vi "RT - DI Status Change.vi"(6 "DI Index":i32, 8 "Error In":errorcluster, 9 "Last Status":bool, 10 "Current Status":bool, 11 "Message Queue":refnum<queue>) -> (0 "Error Out":errorcluster, 2 "Current Status Out":bool, 3 "dup Message Queue":refnum<queue>)   [LabVIEW 2018]
uses:
  Message Queue/Message Cluster.ctl
  Message Queue/Message.ctl
  Controls/Control Mode.ctl
  Controls/DI Status Message.ctl
  Message Queue/Message Queue.lvlib
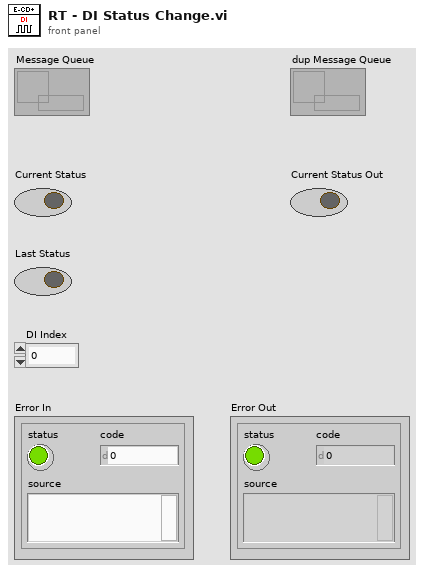
[diagram p1: front panel]
types:
  T1 = typedef "Message Queue.lvlib/Message.ctl" = enum16{"Initialize", "Initialize UI Refs", "Disable Controls", "Enable UI Controls", "Connect RT", "Get Control Mode from RT", "Send Control Mode to UI", "Update Control Mode", "Get Config from RT", "Send Config to UI", "Update Parameters", "Change Parameters", "Calibrate Config", "Update Calibration", "Change Valve State", "Get Valve Status from RT", "Send Valve Status to UI", "Update Valve Status", "Inital UI Values", "Disconnect RT", "Close Connection", "Disconnect UI", "Run Mode", "Stop ALL", "Change Control Mode", "Skid Manual", "Computer Manual", "Step Automated", "Fully Automated", "Reset", "Pumps Command", "Pump State Changed", "Critical Error", "Log-Only Error", "Non-Critical Error", "RT Error", "Update System Status", "Update DI Status", "Clear System Status", "Update Warning", "Clear Warning", "Upate Timeout", "Update Reset Status", "Waiting", "Verify Password", "Manual Cleaning Process", "Update Manual Cleaning Process", "Cal - Body", "Cal - US", "Cal - Update Parameters", "Exit", "---Copy This Frame---"}
  T2 = typedef "Control Mode.ctl" = enum16{"Skid Manual", "Computer Manual", "Step Automated", "Fully Automated"}
  T3 = typedef "DI Status Message.ctl" = cluster{"Message":string, "DI Index #":i32, "Status":bool}
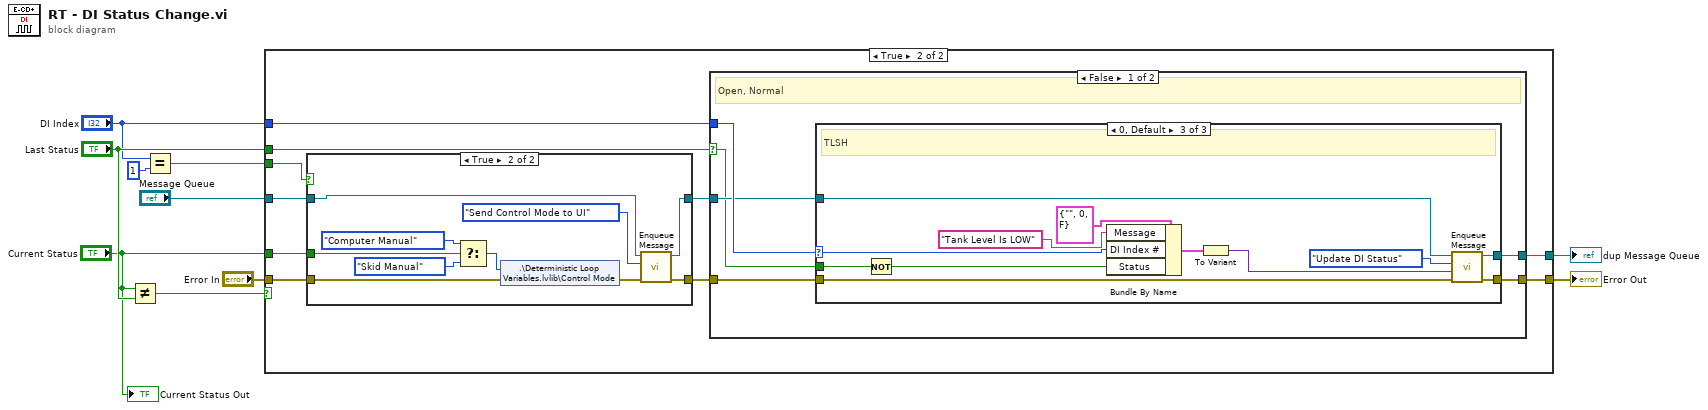
[diagram p0: block diagram]
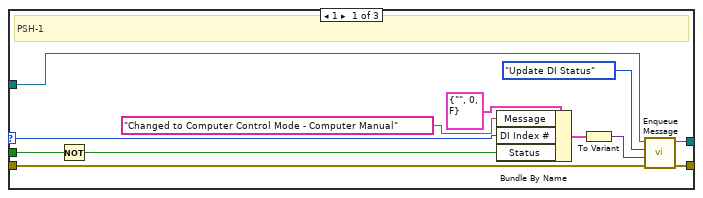
[diagram p4: hidden frame]
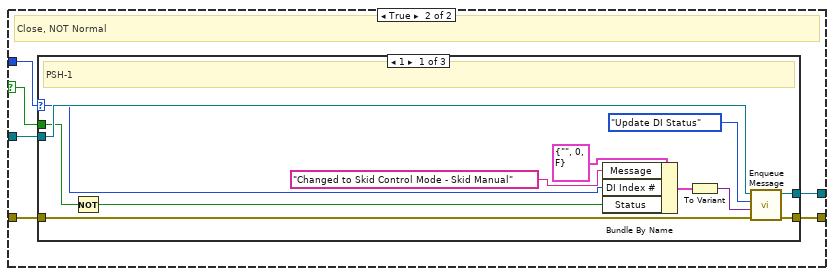
[diagram p6: hidden frame]
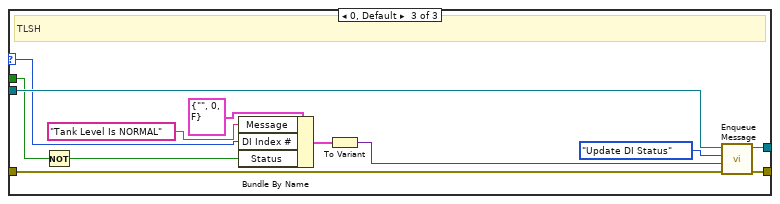
[diagram p8: hidden frame]
diagram:
  n1 = Not Equal?(x="Current Status", y="Last Status") -> (x != y?=w6:bool)
  n2 = Equal?(x="DI Index", y=1) -> (x = y?=w3:bool)
  n3 = case shown="True" w6 {
    tunnel: "Last Status" -> [_ w22]
    tunnel: "DI Index" -> [_ w21]
    tunnel: "Message Queue" -> [w11 w14]
    tunnel: "Error In" -> [w12 w17]
    tunnel: [w12 w20] -> w9
    tunnel: [w11 w19] -> w8
    tunnel: w3 -> [_ w18]
    tunnel: "Current Status" -> [_ w15]
    frame False {
    }
    frame True {
      n4 = case shown="True" w18 {
        tunnel: w17 -> [w24 w30]
        tunnel: [w24 w28] -> w16
        tunnel: w15 -> [_ w34]
        tunnel: w14 -> [w23 w27]
        tunnel: [w23 w26] -> w13
        frame False {
        }
        frame True {
          n5 = Select(t=Control_Mode."Computer Manual" ("Control Mode"), s=w34, f=Control_Mode."Skid Manual") -> (s? t:f=w31:T2)
          n6 = shared-variable ".\\Deterministic Loop Variables.lvlib\\Control Mode"(w31, error in=w30) -> (error out=w29:errorcluster)
          n7 = call "Enqueue Message.vi"("error in (no error)"=w29, "Message"=Message."Send Control Mode to UI", "Message Queue"=w27) -> ("error out"=w28:errorcluster, "dup Message Queue"=w26:refnum<queue>)  [unwired: 7 in]
        }
      }
      n8 = case shown="False" w22 {
        selector: w22 -> [w36 w68]
        tunnel: w13 -> [w39 w71]
        tunnel: w21 -> [w40 w72]
        tunnel: w16 -> [w38 w70]
        tunnel: [w37 w69] -> w20
        tunnel: [w35 w67] -> w19
        frame False {
          # "Open, Normal"
          n9 = case shown="0, Default" w40 {
            selector: w40 -> [w47 _ w61]
            tunnel: w39 -> [w52 w54 w66]
            tunnel: w38 -> [w50 w53 w64]
            tunnel: [w49 w53 w63] -> w37
            tunnel: w36 -> [w46 _ w60]
            tunnel: [w41 w54 w55] -> w35
            frame 1 {
              # "PSH-1"
              n10 = Not(x=w46) -> (.not. x?=w45:bool)
              n11 = Bundle By Name(cluster=T3 {"Message"="", "DI Index #"=0, "Status"=FALSE} ("DI Status Message"), "Message"="Changed to Computer Control Mode - Computer Manual", "DI Index #"=w47, "Status"=w45) -> (w43:T3)
              n12 = To Variant(anything=w43) -> (Variant=w44:variant)
              n13 = call "Enqueue Message.vi"("error in (no error)"=w50, "Message Data"=w44, "Message"=Message."Update DI Status", "Message Queue"=w52) -> ("error out"=w49:errorcluster, "dup Message Queue"=w41:refnum<queue>)  [unwired: 6 in]
            }
            frame 2..22 {
            }
            frame 0, Default {
              # "TLSH"
              n14 = Not(x=w60) -> (.not. x?=w59:bool)
              n15 = Bundle By Name(cluster=T3 {"Message"="", "DI Index #"=0, "Status"=FALSE} ("DI Status Message"), "Message"="Tank Level Is LOW", "DI Index #"=w61, "Status"=w59) -> (w57:T3)
              n16 = To Variant(anything=w57) -> (Variant=w58:variant)
              n17 = call "Enqueue Message.vi"("error in (no error)"=w64, "Message Data"=w58, "Message"=Message."Update DI Status", "Message Queue"=w66) -> ("error out"=w63:errorcluster, "dup Message Queue"=w55:refnum<queue>)  [unwired: 6 in]
            }
          }
        }
        frame True {
          # "Close, NOT Normal"
          n18 = case shown="1" w72 {
            selector: w72 -> [w80 _ w93]
            tunnel: w71 -> [w84 w86 w98]
            tunnel: w70 -> [w74 w85 w96]
            tunnel: [w82 w85 w95] -> w69
            tunnel: w68 -> [w79 _ w92]
            tunnel: [w75 w86 w87] -> w67
            frame 1 {
              # "PSH-1"
              n19 = Not(x=w79) -> (.not. x?=w73:bool)
              n20 = Bundle By Name(cluster=T3 {"Message"="", "DI Index #"=0, "Status"=FALSE} ("DI Status Message"), "Message"="Changed to Skid Control Mode - Skid Manual", "DI Index #"=w80, "Status"=w73) -> (w77:T3)
              n21 = To Variant(anything=w77) -> (Variant=w78:variant)
              n22 = call "Enqueue Message.vi"("error in (no error)"=w74, "Message Data"=w78, "Message"=Message."Update DI Status", "Message Queue"=w84) -> ("error out"=w82:errorcluster, "dup Message Queue"=w75:refnum<queue>)  [unwired: 6 in]
            }
            frame 2..22 {
            }
            frame 0, Default {
              # "TLSH"
              n23 = Not(x=w92) -> (.not. x?=w91:bool)
              n24 = Bundle By Name(cluster=T3 {"Message"="", "DI Index #"=0, "Status"=FALSE} ("DI Status Message"), "Message"="Tank Level Is NORMAL", "DI Index #"=w93, "Status"=w91) -> (w89:T3)
              n25 = To Variant(anything=w89) -> (Variant=w90:variant)
              n26 = call "Enqueue Message.vi"("error in (no error)"=w96, "Message Data"=w90, "Message"=Message."Update DI Status", "Message Queue"=w98) -> ("error out"=w95:errorcluster, "dup Message Queue"=w87:refnum<queue>)  [unwired: 6 in]
            }
          }
        }
      }
    }
  }
  "Error Out" <- w9
  "dup Message Queue" <- w8
  "Current Status Out" <- "Current Status"
